vi "get_sre.vi"(8 "error in (no error)":errorcluster, 11 "VISA Refnum in":refnum<visa-resource-name>) -> (0 "error out":errorcluster, 2 "SRE":string, 3 "VISA Refnum out":refnum<visa-resource-name>)   [LabVIEW 2018, in "Aim-TTi PL303-P.lvlib"]
uses:
  <instrlib>/Aim-TTi PL303-P/Aim-TTi PL303-P.lvlib
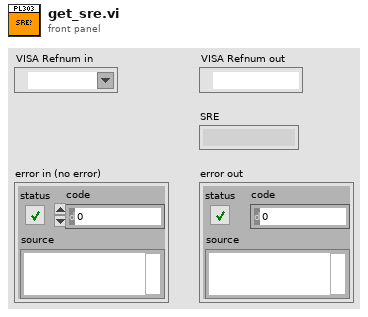
[diagram p1: front panel]
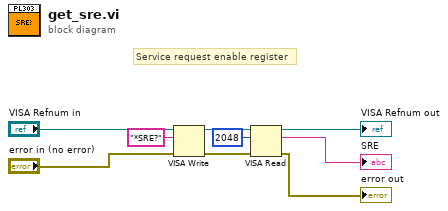
[diagram p0: block diagram]
diagram:
  # "Service request enable register"
  n1 = VISA Write(VISA resource name="VISA Refnum in", write buffer="*SRE?", error in (no error)="error in (no error)") -> (VISA resource name out=w1:refnum<visa-resource-name>, error out=w2:errorcluster)  [unwired: 1 out]
  n2 = VISA Read(VISA resource name=w1, byte count=u32 2048, error in (no error)=w2) -> (VISA resource name out=→"VISA Refnum out":refnum<visa-resource-name>, read buffer=→"SRE":string, error out=→"error out":errorcluster)  [unwired: 1 out]
